vi "REceptorUSART V2.vi"() -> ()   [LabVIEW 2015]
uses:
  <vilib>/Instr/_visa.llb/Select Event Type.ctl
  <vilib>/Instr/_visa.llb/VISA Configure Serial Port (Instr).vi
panel:
  out "Waveform":waveform(dbl)(graph)
  out "Iluminancia":i32(graph)
  out "Humedades y Potencia lumínica":cluster{"f":dbl, "f":i32}(graph)
  in  "Plot Humedad Tierra":bool
  in  "Plot Potencia Luminica":bool
  in  "Plot Humedad Relativa":bool
  out "Humedad Relativa %":dbl(knob) scale=0.0..100.0
  out "Humedad Tierra %":dbl(knob) scale=0.0..100.0
  out "Iluminancia LUX":i32(knob) scale=10.0..100000.0
  in  "Plot MCP9808":bool
  in  "Plot Temp DHT22":bool
  in  "Plot Analog Temp":bool
  out "Termometro I2C MCP9808":dbl(slide) scale=-20.0..50.0
  out "Temp Analog":i16(slide) caption="Thermometer" scale=-20.0..50.0
  out "Temp Digital":i16(slide) caption="Thermometer" scale=-20.0..50.0
  out "Temperaturas":cluster{i32, "f":i32, "f":i32}(graph)
  in  "Solicitar Muestras":bool
  out "ON":bool
  in  "stop":bool
  out "read buffer":string
  in  "PORT COM IMPUT":refnum<visa-resource-name>
  # "DHT22 Sensor"
  # "Control Panel"
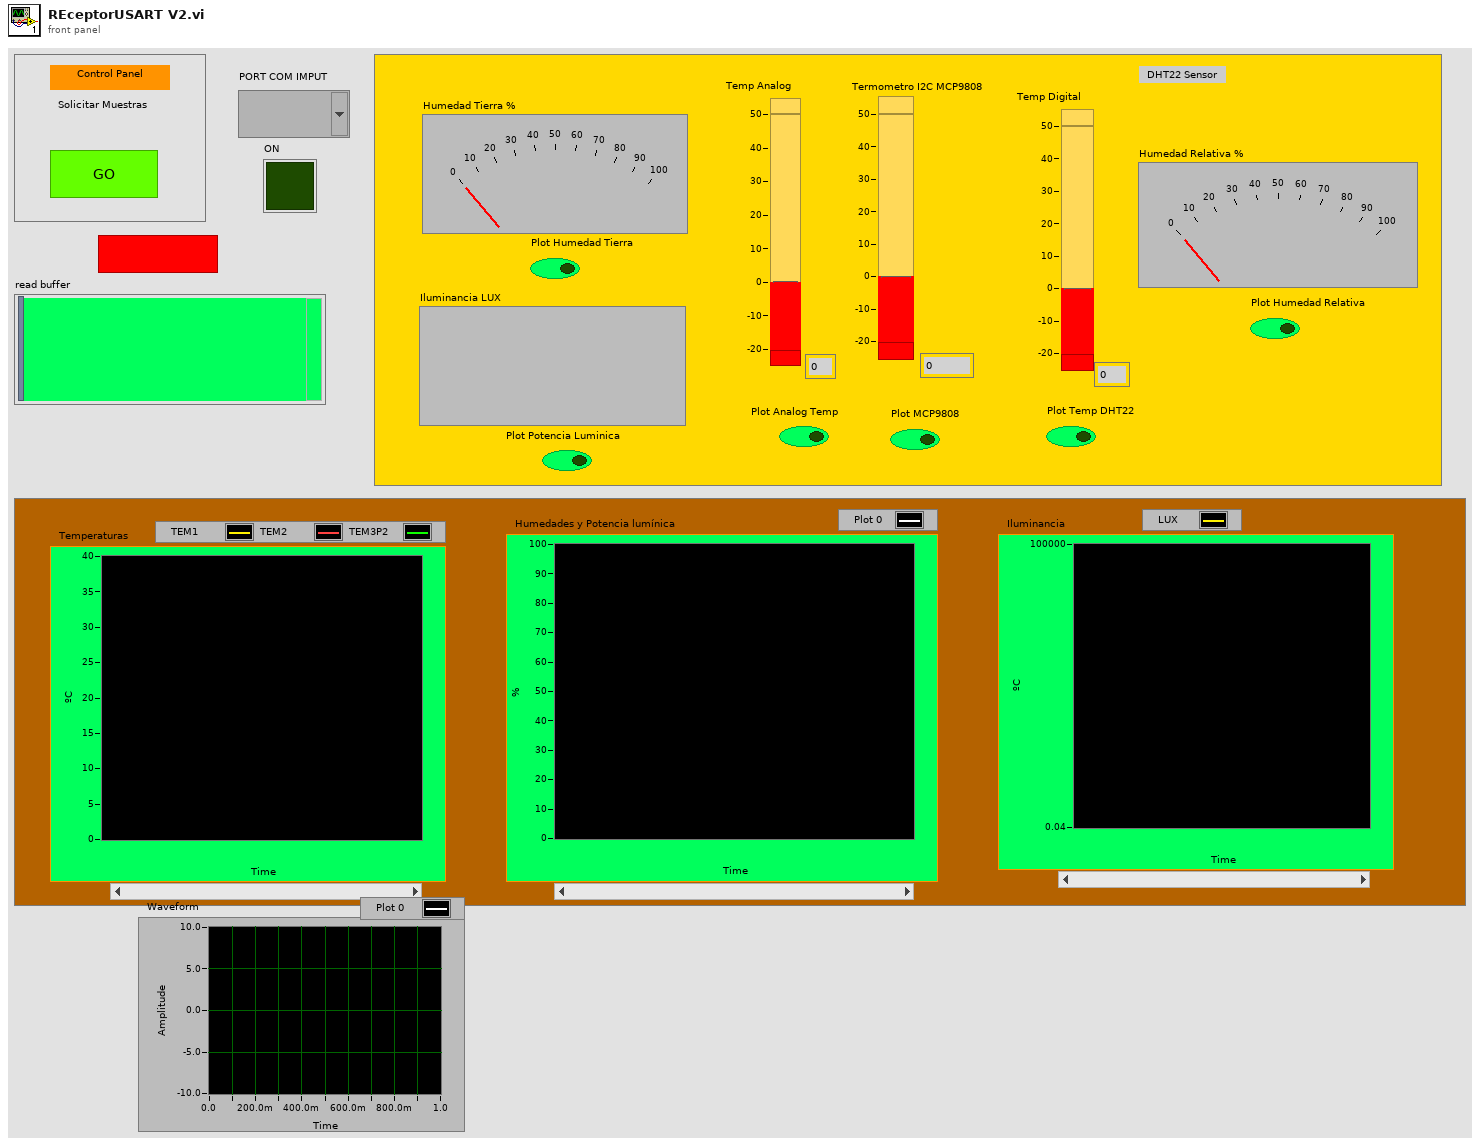
[diagram p1: front panel]
types:
  T1 = typedef "Select Event Type.ctl" = u32
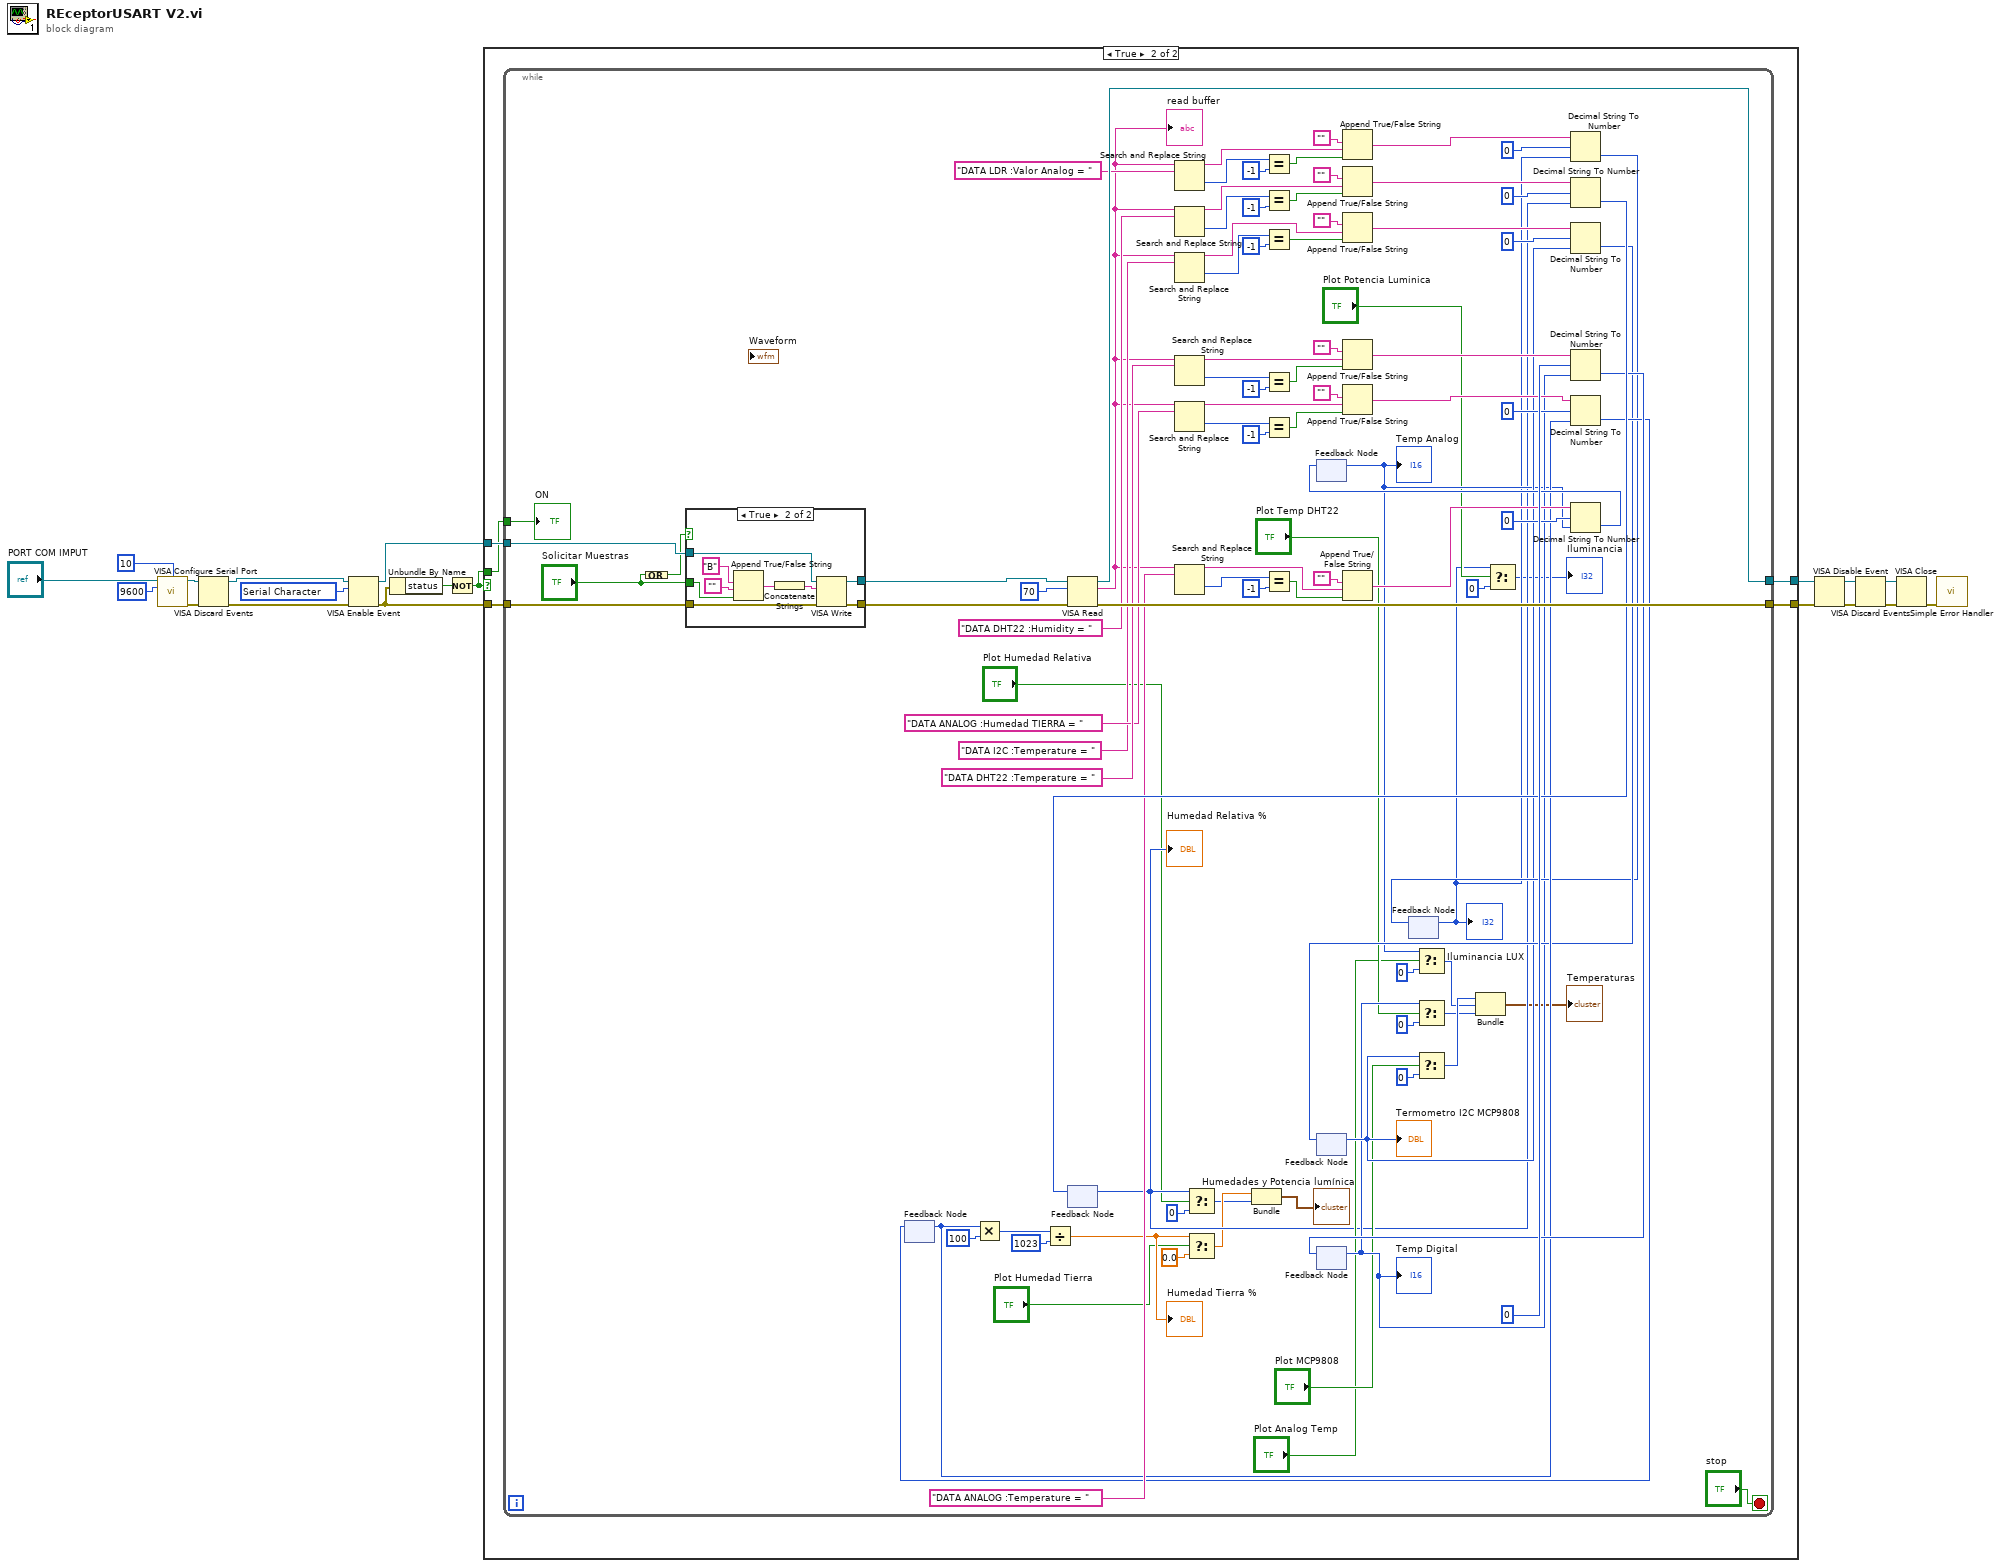
[diagram p0: block diagram]
diagram:
  w16 = T1 1073684533 items=["Service Request"=1073684491, "Trigger"=3221168138, "Clear"=1073684493, "VXI Signal"=1073684512, "VXI/VME Interrupt"=3221168161, "VXI/VME Sysfail"=1073684509, "VXI/VME Sysreset"=1073684510, "GPIB CIC"=1073684498, "GPIB Talk"=1073684499, "GPIB Listen"=1073684500, "PXI Interrupt"=1073684514, "Serial Break"=1073684515, "Serial TermChar"=1073684516, "Serial CTS"=1073684521, "Serial DSR"=1073684522, "Serial DCD"=1073684524, "Serial RI"=1073684526, "Serial Character"=1073684533, "USB Interrupt"=1073684535, "All Enabled"=1073709055] ("Event Type")
  n1 = call-poly "VISA Configure Serial Port"("VISA resource name"="PORT COM IMPUT", "termination char\n(0xA = '\\n' = LF)"=u8 10 ("termination char\n(0xA = '\\n' = LF)"), "baud rate (9600)"=u32 9600) -> ("VISA resource name out"=w5:refnum<visa-resource-name>, "error out"=w4:errorcluster)  [unwired: 11 in]
  n2 = VISA Discard Events(8:w4, 11:w5) -> (0:w17:errorcluster, 3:w18:refnum<visa-resource-name>)  [unwired: 2 in]
  n3 = VISA Enable Event(8:w17, 10:w16, 11:w18) -> (0:w2:errorcluster, 3:w3:refnum<visa-resource-name>)  [unwired: 1 in]
  n4 = Unbundle By Name(w2) -> ("status"=w15:bool)
  n5 = Not(x=w15) -> (.not. x?=w1:bool)
  n6 = case shown="True" w1 {
    tunnel: w2 -> [w21 w26]
    tunnel: w3 -> [w20 w25]
    tunnel: w1 -> [_ w24]
    tunnel: [w21 w22] -> w10
    tunnel: [w20 w23] -> w9
    frame False {
    }
    frame True {
      n7 = while {
        tunnel: w26 -> [w118]
        tunnel: w25 -> [w117]
        tunnel: w24 -> [w120]
        tunnel: [w122] -> w23
        tunnel: [w121] -> w22
        stop <- "stop" stop-if-true
        n8 = Compound Arithmetic op=OR("Solicitar Muestras") -> (w114:bool)
        n9 = case shown="True" w114 {
          tunnel: w117 -> [w124 w133]
          tunnel: w118 -> [w123 w132]
          tunnel: [w124 w131] -> w28
          tunnel: [w123 w130] -> w27
          tunnel: "Solicitar Muestras" -> [_ w127]
          frame False {
          }
          frame True {
            n10 = Append True/False String(1:w127, 2:"", 3:"B") -> (0:w128:string)  [unwired: 1 in]
            n11 = Concatenate Strings(w128) -> (w129:string)
            n12 = VISA Write(VISA resource name=w133, write buffer=w129, error in (no error)=w132) -> (VISA resource name out=w131:refnum<visa-resource-name>, error out=w130:errorcluster)  [unwired: 1 out]
          }
        }
        n13 = feedback #1() -> (w70:i32)  [unwired: 1 in]
        n14 = Multiply(x=w70, y=100) -> (x*y=w69:i32)
        n15 = Divide(x=w69, y=1023) -> (x/y=w41:dbl)
        "Humedad Tierra %" <- w41
        n16 = VISA Read(VISA resource name=w28, byte count=u32 70, error in (no error)=w27) -> (VISA resource name out=w122:refnum<visa-resource-name>, read buffer=w57:string, error out=w121:errorcluster)  [unwired: 1 out]
        "read buffer" <- w57
        n17 = feedback #2() -> (w42:i32)  [unwired: 1 in]
        "Humedad Relativa %" <- w42
        n18 = Search and Replace String(input string=w57, search string="DATA LDR :Valor Analog = ") -> (result string=w107:string, offset past replacement=w109:i32)  [unwired: 6 in, 2 out]
        n19 = Search and Replace String(input string=w57, search string="DATA DHT22 :Humidity = ") -> (result string=w101:string, offset past replacement=w103:i32)  [unwired: 6 in, 2 out]
        n20 = Search and Replace String(input string=w57, search string="DATA I2C :Temperature = ") -> (result string=w63:string, offset past replacement=w65:i32)  [unwired: 6 in, 2 out]
        n21 = Search and Replace String(input string=w57, search string="DATA DHT22 :Temperature = ") -> (result string=w84:string, offset past replacement=w86:i32)  [unwired: 6 in, 2 out]
        n22 = Search and Replace String(input string=w57, search string="DATA ANALOG :Humedad TIERRA = ") -> (result string=w76:string, offset past replacement=w78:i32)  [unwired: 6 in, 2 out]
        n23 = Search and Replace String(input string=w57, search string="DATA ANALOG :Temperature = ") -> (result string=w93:string, offset past replacement=w95:i32)  [unwired: 6 in, 2 out]
        n24 = Select(t=w42, s="Plot Humedad Relativa", f=0) -> (s? t:f=w34:i32)
        n25 = Select(t=w41, s="Plot Humedad Tierra", f=0.0) -> (s? t:f=w35:dbl)
        n26 = Bundle("f"=w35, "f"=w34) -> (→"Humedades y Potencia lumínica":cluster{"f":dbl, "f":i32})  [unwired: 1 in]
        n27 = Equal?(x=w109, y=-1) -> (x = y?=w105:bool)
        n28 = Equal?(x=w103, y=-1) -> (x = y?=w99:bool)
        n29 = Equal?(x=w65, y=-1) -> (x = y?=w62:bool)
        n30 = Equal?(x=w86, y=-1) -> (x = y?=w83:bool)
        n31 = Equal?(x=w78, y=-1) -> (x = y?=w75:bool)
        n32 = Equal?(x=w95, y=-1) -> (x = y?=w91:bool)
        n33 = feedback #3() -> (w50:i32)  [unwired: 1 in]
        "Temp Analog" <- w50
        n34 = feedback #4() -> (w54:i32)  [unwired: 1 in]
        "Termometro I2C MCP9808" <- w54
        n35 = feedback #5() -> (w51:i32)  [unwired: 1 in]
        "Temp Digital" <- w51
        n36 = Append True/False String(1:w105, 2:w107, 3:"") -> (0:w88:string)  [unwired: 1 in]
        n37 = Append True/False String(1:w99, 2:w101, 3:"") -> (0:w98:string)  [unwired: 1 in]
        n38 = Append True/False String(1:w62, 2:w63, 3:"") -> (0:w61:string)  [unwired: 1 in]
        n39 = Append True/False String(1:w83, 2:w84, 3:"") -> (0:w80:string)  [unwired: 1 in]
        n40 = Append True/False String(1:w75, 2:w76, 3:"") -> (0:w74:string)  [unwired: 1 in]
        n41 = Append True/False String(1:w91, 2:w93, 3:"") -> (0:w89:string)  [unwired: 1 in]
        n42 = feedback #6() -> (w33:i32)  [unwired: 1 in]
        "Iluminancia LUX" <- w33
        n43 = Select(t=w50, s="Plot Analog Temp", f=0) -> (s? t:f=w53:i32)
        n44 = Select(t=w51, s="Plot Temp DHT22", f=0) -> (s? t:f=w52:i32)
        n45 = Select(t=w54, s="Plot MCP9808", f=0) -> (s? t:f=w55:i32)
        n46 = Bundle("f"=w55, "f"=w53, "f"=w52) -> (→"Temperaturas":cluster{"f":i32, "f":i32, "f":i32})  [unwired: 1 in]
        n47 = Select(t=w33, s="Plot Potencia Luminica", f=0) -> (s? t:f=→"Iluminancia":i32)
        n48 = Decimal String To Number(string=w88, offset=0, default (0L)=w33) -> (number=w56:i32)  [unwired: 1 out]
        n49 = feedback-in #6(w56) -> ()
        n50 = Decimal String To Number(string=w98, offset=0, default (0L)=w42) -> (number=w97:i32)  [unwired: 1 out]
        n51 = feedback-in #2(w97) -> ()
        n52 = Decimal String To Number(string=w61, offset=0, default (0L)=w54) -> (number=w59:i32)  [unwired: 1 out]
        n53 = feedback-in #4(w59) -> ()
        n54 = Decimal String To Number(string=w80, offset=0, default (0L)=w51) -> (number=w96:i32)  [unwired: 1 out]
        n55 = feedback-in #5(w96) -> ()
        n56 = Decimal String To Number(string=w74, offset=0, default (0L)=w70) -> (number=w72:i32)  [unwired: 1 out]
        n57 = feedback-in #1(w72) -> ()
        n58 = Decimal String To Number(string=w89, offset=0, default (0L)=w50) -> (number=w87:i32)  [unwired: 1 out]
        n59 = feedback-in #3(w87) -> ()
        "ON" <- w120
      }
    }
  }
  n60 = VISA Disable Event(8:w10, 11:w9) -> (0:w11:errorcluster, 3:w12:refnum<visa-resource-name>)  [unwired: 2 in]
  n61 = VISA Discard Events(8:w11, 11:w12) -> (0:w14:errorcluster, 3:w13:refnum<visa-resource-name>)  [unwired: 2 in]
  n62 = VISA Close(VISA resource name=w13, error in (no error)=w14) -> (error out=w7:errorcluster)
  n63 = call <vilib>:"Simple Error Handler.vi"("error in (no error)"=w7) -> ()  [unwired: 1 in, 8 out]
